vi "svfa_Average Spectrum (real) No State.vi"(0 "spectrum":cluster{"f0":dbl, "df":dbl, "spectrum":dbl[]} {"spectrum" format="%.2p"; "df" format="%.2p"; "f0" format="%.2p"}, 1 "processing control":T1(ring), 7 "averaging parameters":T3={"averaging mode"=enum."No averaging", "weighting mode"=enum."Linear", "number of averages"=10, "linear mode"=enum."Auto restart"}, 11 "error in (no error)":errorcluster, 12 "averaging state info in":T2={"complex FFT"=[], "real FFT"=[], "f0"=0.0, "df"=0.0, "averages completed"=0.0, "averaging parameters"={"averaging mode"=enum."No averaging", "weighting mode"=enum."Linear", "number of averages"=10, "linear mode"=enum."Auto restart"}} {"averages completed" format="%.2f"; "df" format="%.2f"; "f0" format="%.2f"; "real FFT" format="%.2f"; "complex FFT" format="%.2f"}) -> (4 "average spectrum":cluster{"f0":dbl, "df":dbl, "spectrum":dbl[]} {"spectrum" format="%.2p"; "df" format="%.2p"; "f0" format="%.2p"}, 6 "new spectrum ready":bool, 8 "averaging done":bool, 10 "averages completed":dbl, 14 "averaging state info out":T2={"complex FFT"=[], "real FFT"=[], "f0"=0.0, "df"=0.0, "averages completed"=0.0, "averaging parameters"={"averaging mode"=enum."No averaging", "weighting mode"=enum."Linear", "number of averages"=10, "linear mode"=enum."Auto restart"}} {"averages completed" format="%.2f"; "df" format="%.2f"; "f0" format="%.2f"; "real FFT" format="%.2f"; "complex FFT" format="%.2f"}, 15 "error out":errorcluster)   [LabVIEW 2017]
uses:
  <vilib>/addons/_NISVFA/_Shared subVIs/Spectrum Averaging/svfa_Average Array (real) No State.vi
  <vilib>/addons/_NISVFA/_Shared subVIs/Spectrum Averaging/svfa_No Average Array (real).vi
  <vilib>/addons/_NISVFA/_Shared subVIs/Spectrum Averaging/svfa_Average Array (real).vi
  <vilib>/addons/_NISVFA/_Shared subVIs/Spectrum Averaging/svfa_Peak Hold Array.vi
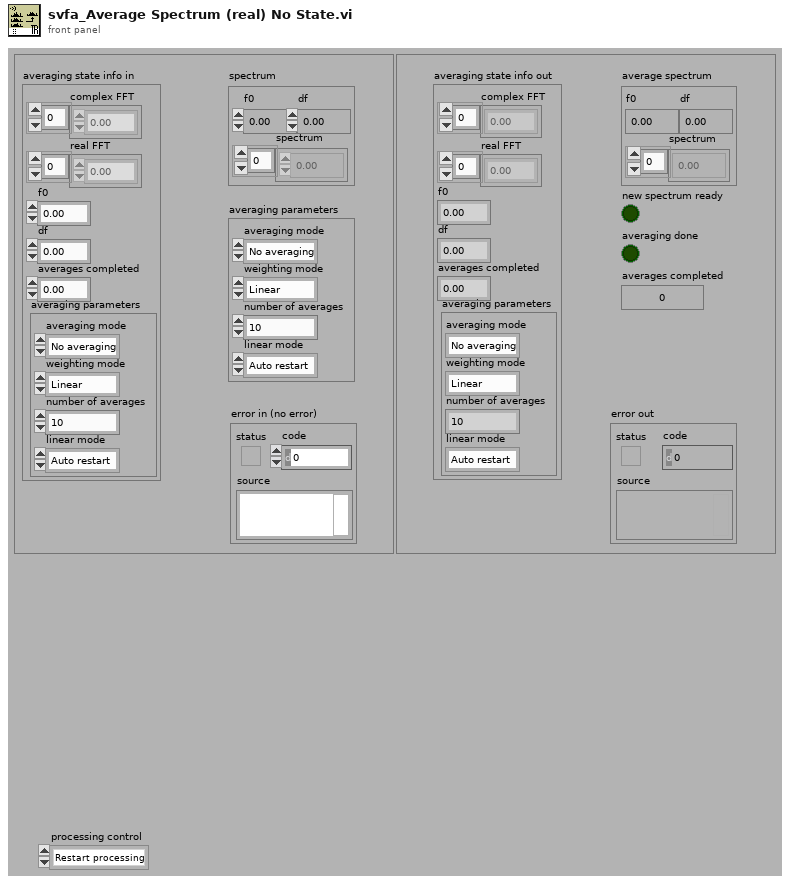
[diagram p1: front panel]
types:
  T1 = enum16{"Restart processing", "Continue processing", "Skip processing"}
  T2 = cluster{"complex FFT":cdb[], "real FFT":dbl[], "f0":dbl, "df":dbl, "averages completed":dbl, "averaging parameters":cluster{"averaging mode":enum16{"No averaging", "Vector averaging", "RMS averaging", "Peak hold"}, "weighting mode":enum16{"Linear", "Exponential"}, "number of averages":u32, "linear mode":enum16{"One shot", "Auto restart"}}}
  T3 = cluster{"averaging mode":enum16{"No averaging", "Vector averaging", "RMS averaging", "Peak hold"}, "weighting mode":enum16{"Linear", "Exponential"}, "number of averages":u32, "linear mode":enum16{"One shot", "Auto restart"}}
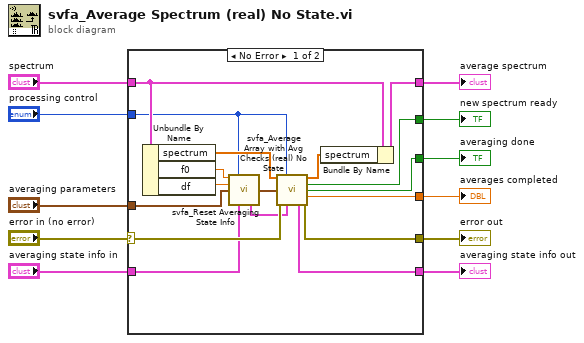
[diagram p0: block diagram]
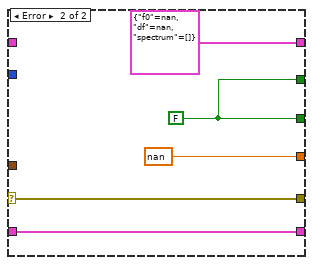
[diagram p2: hidden frame]
diagram:
  n1 = case shown="No Error" "error in (no error)" {
    selector: "error in (no error)" -> [w15 w33]
    tunnel: [w23 w33] -> w4
    tunnel: "averaging parameters" -> [w21 _]
    tunnel: [w27 w30] -> w5
    tunnel: [w28 w30] -> w3
    tunnel: [w26 nan ("f0")] -> w11
    tunnel: "spectrum" -> [w16 _]
    tunnel: "averaging state info in" -> [w14 w32]
    tunnel: [w25 w32] -> w2
    tunnel: [w24 cluster{"f0":dbl, "df":dbl, "spectrum":dbl[]} {"f0"=nan, "df"=nan, "spectrum"=[]} ("dup spectrum")] -> w10
    tunnel: "processing control" -> [w12 _]
    frame No Error {
      n2 = Unbundle By Name(w16) -> ("spectrum"=w19:dbl[], "f0"=w18:dbl, "df"=w17:dbl)
      n3 = call <vilib>:"svfa_Reset Averaging State Info.vi"("f0"=w18, "processing control"=w12, "df"=w17, "averaging parameters"=w21, "averaging state info in"=w14) -> ("dup averaging parameters"=w20:T3, "averaging state info out"=w13:T2)  [unwired: 9 in]
      n4 = call <vilib>:"svfa_Average Array with Avg Checks (real) No State.vi"("spectrum"=w19, "processing control"=w12, "averaging parameters"=w20, "error in"=w15, "averaging state info"=w13) -> ("avg spectrum"=w22:dbl[], "new spectrum ready"=w28:bool, "averaging done"=w27:bool, "averages completed"=w26:dbl, "averaging state info"=w25:T2, "error out"=w23:errorcluster)  [unwired: 5 in]
      n5 = Bundle By Name(cluster=w16, "spectrum"=w22) -> (w24:cluster{"f0":dbl, "df":dbl, "spectrum":dbl[]})
    }
    frame Error {
      w30 = FALSE
    }
  }
  "averages completed" <- w11
  "average spectrum" <- w10
  "averaging done" <- w5
  "error out" <- w4
  "new spectrum ready" <- w3
  "averaging state info out" <- w2
